vi "state.vi"(4 "reference":refnum<vi>, 6 "temperatura":dbl, 7 "danger":dbl, 8 "warning":dbl) -> (0 "string":string, 1 "DANGER":bool, 2 "WARNING":bool, 3 "NORMAL":bool)   [LabVIEW 2021]
panel:
  out "Array":u8[](array[numeric])
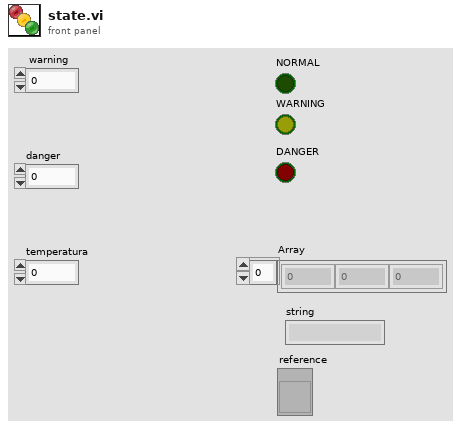
[diagram p1: front panel]
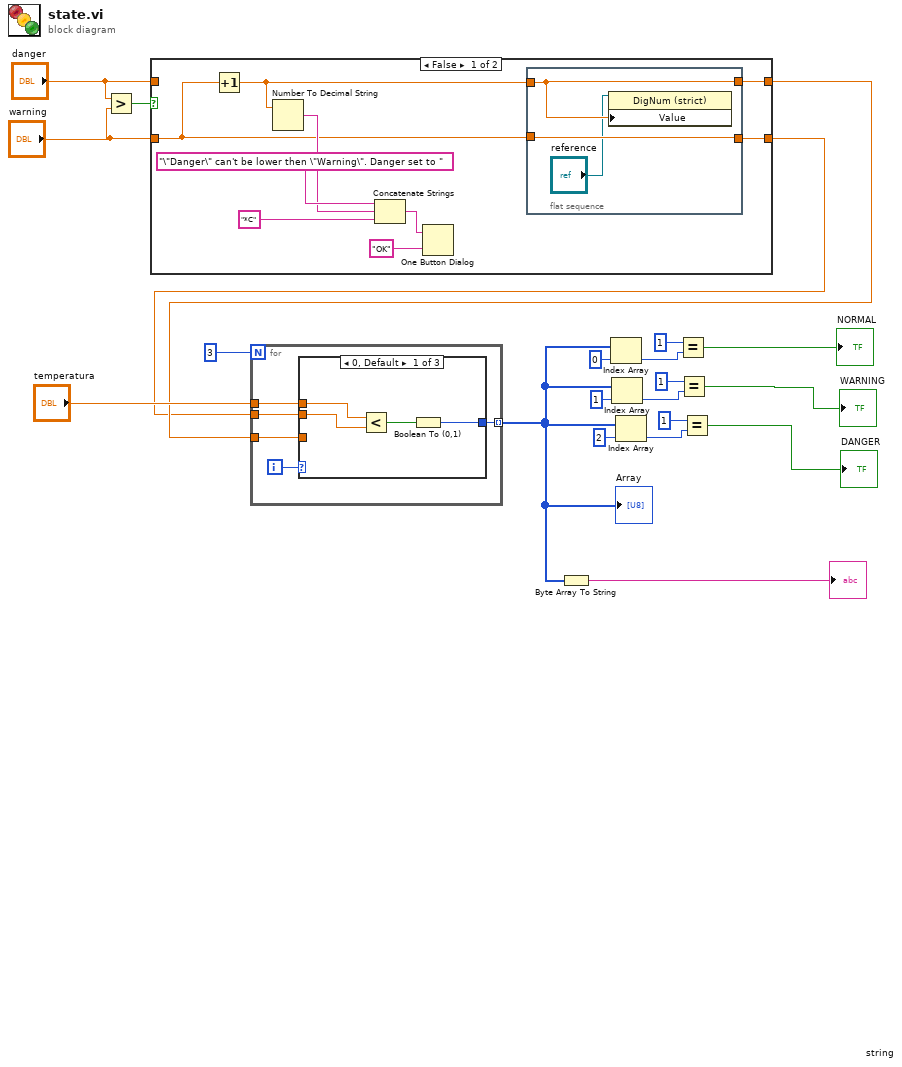
[diagram p0: block diagram]
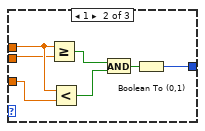
[diagram p3: hidden frame]
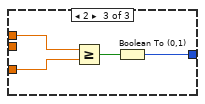
[diagram p4: hidden frame]
diagram:
  n1 = Greater?(x="danger", y="warning") -> (0:w5:bool)
  n2 = case shown="False" w5 {
    tunnel: [w25 w35] -> w2
    tunnel: "danger" -> [_ w35]
    tunnel: [w24 w34] -> w1
    tunnel: "warning" -> [w23 w34]
    frame False {
      n3 = Increment(x=w23) -> (x+1=w22:dbl)
      n4 = Number To Decimal String(number=w22) -> (decimal integer string=w28:string)  [unwired: 1 in]
      n5 = Concatenate Strings("\"Danger\" can't be lower then \"Warning\". Danger set to " ("message"), w28, "*C" ("string")) -> (w27:string)
      n6 = One Button Dialog(message=w27, button name ("OK")="OK") -> ()  [unwired: 1 out]
      n7 = flat-sequence {
        tunnel: w22 -> [w32]
        tunnel: [w32] -> w25
        tunnel: w23 -> [w33]
        tunnel: [w33] -> w24
        frame #0 {
          n8 = property class="DigNum (strict)"(reference="reference", "Value"=w32) -> ()  [unwired: 1 in, 2 out]
        }
      }
    }
    frame True {
    }
  }
  n9 = for {
    N: 3 -> [_]
    tunnel: "temperatura" -> [w40]
    tunnel: w1 -> [w39]
    tunnel: w2 -> [w38]
    tunnel: [w36] -> w6 mode=indexing
    i -> [w37]
    n10 = case shown="0, Default" w37 {
      tunnel: w40 -> [w43 w48 w54]
      tunnel: w39 -> [w42 w47 _]
      tunnel: [w41 w45 w52] -> w36
      tunnel: w38 -> [_ w46 w53]
      frame 0, Default {
        n11 = Less?(x=w43, y=w42) -> (x < y?=w44:bool)
        n12 = Boolean To (0,1)(Boolean=w44) -> (0, 1=w41:i16)
      }
      frame 1 {
        n13 = Greater Or Equal?(x=w48, y=w47) -> (x >= y?=w49:bool)
        n14 = Less?(x=w48, y=w46) -> (x < y?=w50:bool)
        n15 = And(x=w49, y=w50) -> (x .and. y?=w51:bool)
        n16 = Boolean To (0,1)(Boolean=w51) -> (0, 1=w45:i16)
      }
      frame 2 {
        n17 = Greater Or Equal?(x=w54, y=w53) -> (x >= y?=w55:bool)
        n18 = Boolean To (0,1)(Boolean=w55) -> (0, 1=w52:i16)
      }
    }
  }
  "Array" <- w6
  n19 = Byte Array To String(unsigned byte array=w6) -> (string=→"string":string)
  n20 = Index Array(array=w6, index=0) -> (element=w12:i16)
  n21 = Index Array(array=w6, index=1) -> (element=w15:i16)
  n22 = Index Array(array=w6, index=2) -> (element=w16:i16)
  n23 = Equal?(x=i8 1, y=w12) -> (x = y?=→"NORMAL":bool)
  n24 = Equal?(x=i8 1, y=w15) -> (x = y?=→"WARNING":bool)
  n25 = Equal?(x=i8 1, y=w16) -> (x = y?=→"DANGER":bool)
